vi "02-旋转样品杆控制上位机顺时针归零.vi"() -> ()   [LabVIEW 2017]
uses:
  <vilib>/Instr/_visa.llb/VISA Configure Serial Port (Instr).vi
panel:
  out "逆时针":bool
  out "顺时针":bool
  out "转动角度命令字符串":string
  out "脉冲字符串":string
  out "脉冲数":u32
  out "归零命令字符串":string
  out "频率字符串":string
  out "频率":u32
  in  "停止运动中的电机":bool
  out "转角相对位置":dbl(knob) scale=0.0..360.0
  in  "电机转速设定":dbl(knob)=10.0 min=0.1 max=10.0 scale=0.1..10.0 scale format="%#_2g"
  in  "转动到设定值":bool
  in  "零点归位":bool
  out "样品杆实际值":dbl(slide) scale=-540.0..540.0 scale format="%.2f"
  in  "停止上位机软件系统":bool
  out "波形图表":cluster{"样品杆设定值":dbl, dbl}(graph)
  in  "旋转样品杆控制端口":refnum<visa-resource-name>
  in  "样品杆设定值":dbl(slide) min=-540.0 max=540.0 scale=-540.0..540.0 scale format="%.2g"
  # "旋转样品杆控制测试程序"
  # "转角绝对位置"
  # "样品杆转动位置曲线"
  # "顺时针"
  # "1"
  # "首先要进行零点归位"
  # "逆时针"
  # "转角相对位置"
  # "电机转速设定"
  # "（度/秒）"
  # "（度）"
  # "（度）"
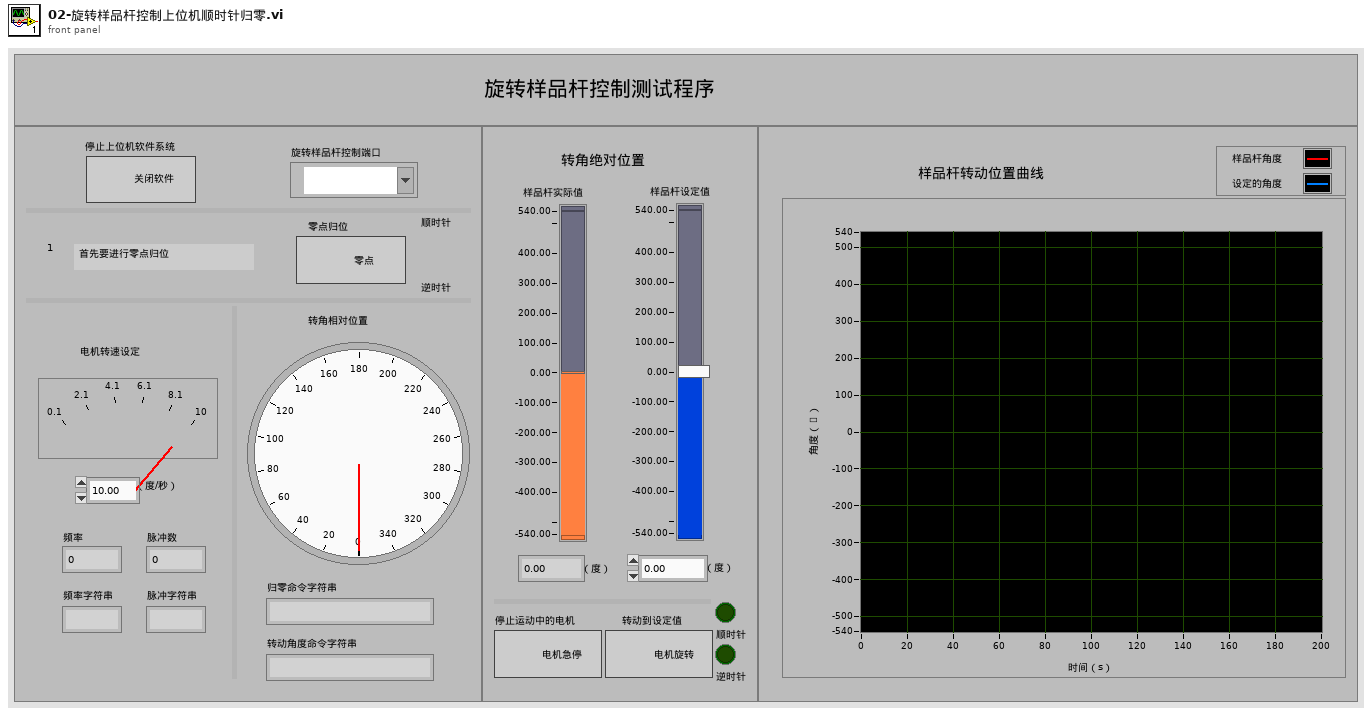
[diagram p1: front panel]
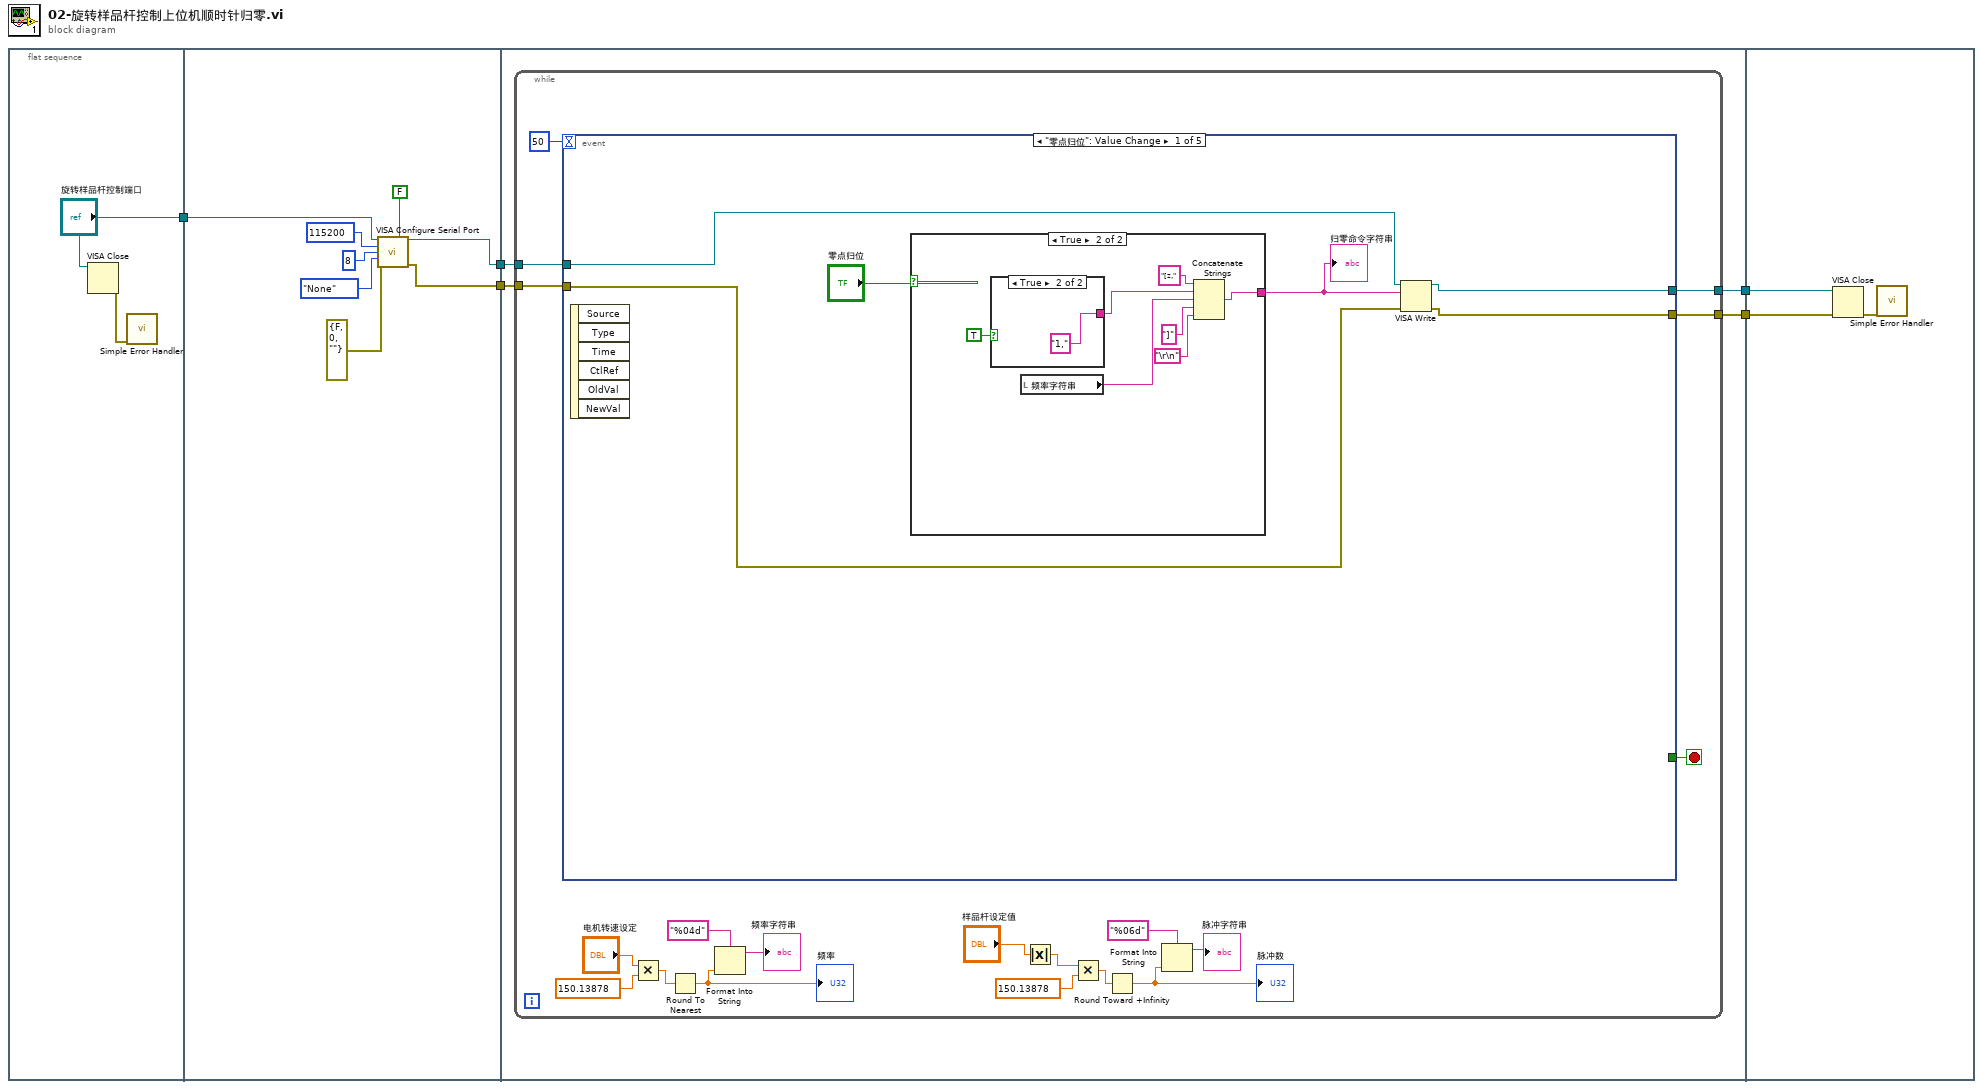
[diagram p0: block diagram]
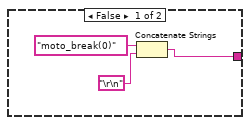
[diagram p2: hidden frame]
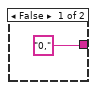
[diagram p3: hidden frame]
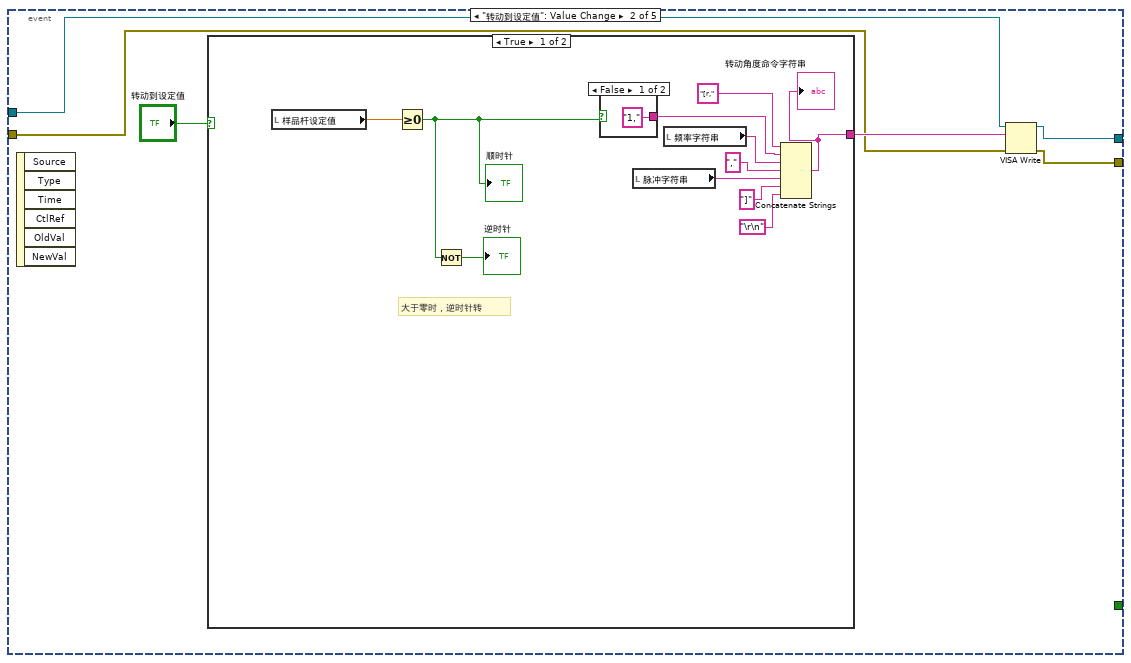
[diagram p4: hidden frame]
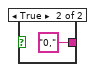
[diagram p5: hidden frame]
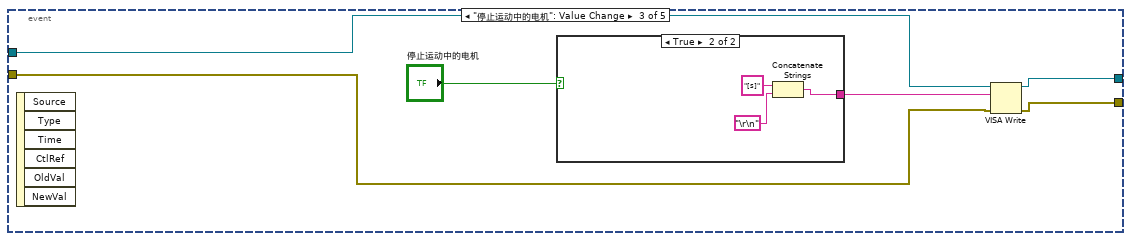
[diagram p7: hidden frame]
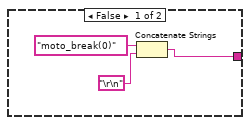
[diagram p8: hidden frame]
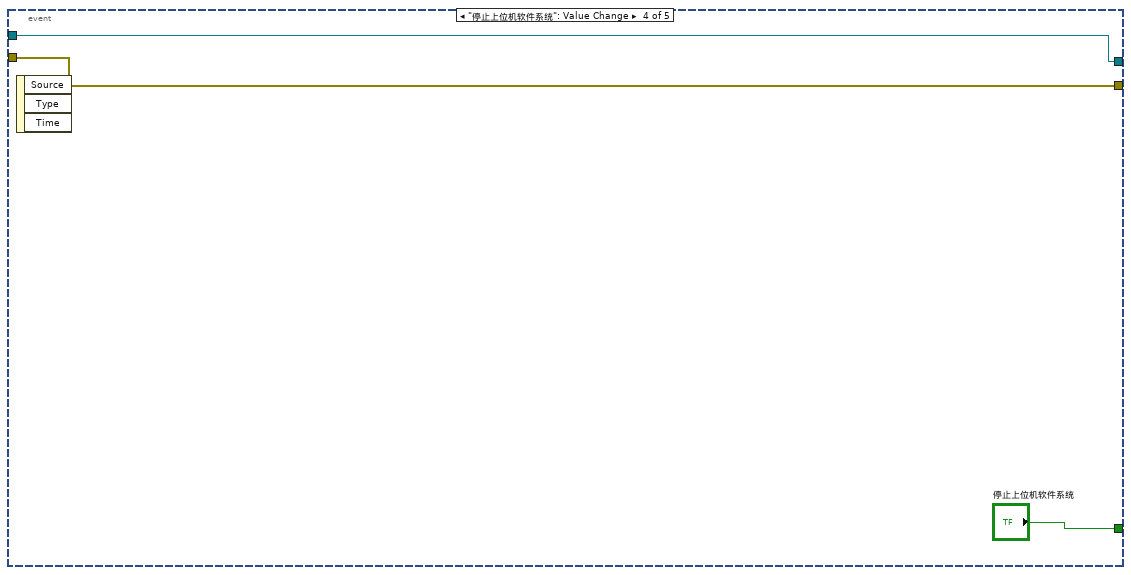
[diagram p9: hidden frame]
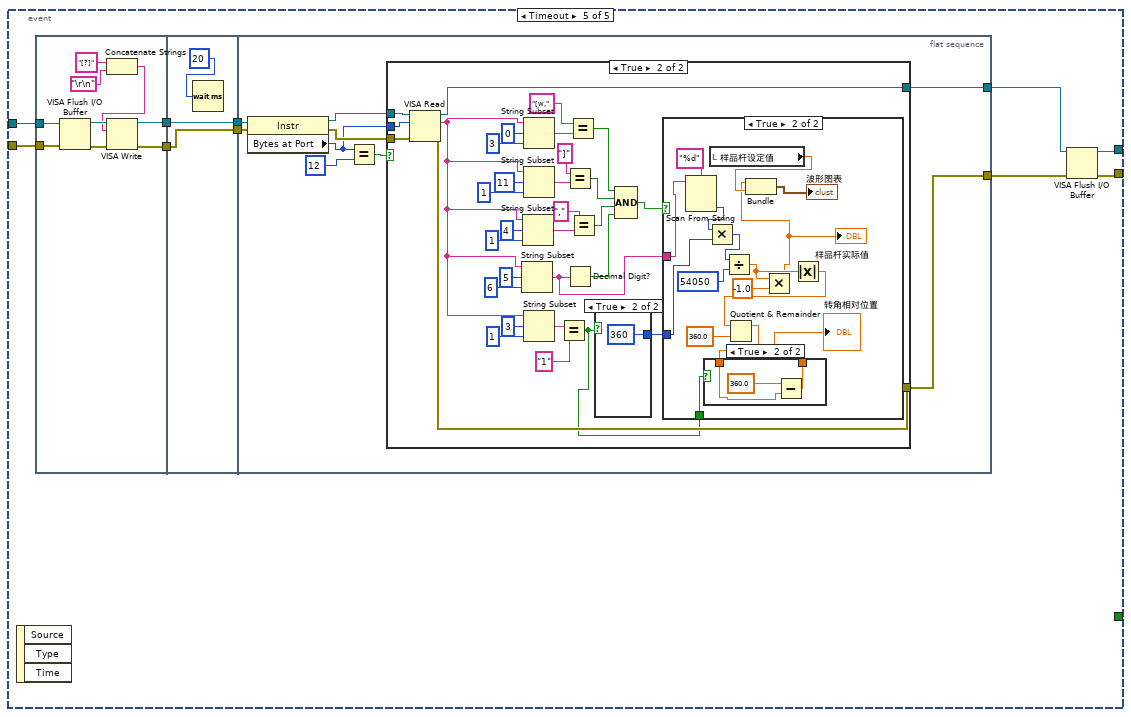
[diagram p10: hidden frame]
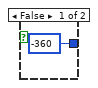
[diagram p12: hidden frame]
diagram:
  n1 = flat-sequence {
    tunnel: ["旋转样品杆控制端口"] -> w1
    tunnel: [w10] -> w3
    tunnel: [w9] -> w2
    tunnel: w1 -> [w8]
    tunnel: [w19] -> w5
    tunnel: [w18] -> w4
    tunnel: w3 -> [w17]
    tunnel: w2 -> [w16]
    tunnel: w5 -> [w180]
    tunnel: w4 -> [w178]
    frame #0 {
      n2 = VISA Close(VISA resource name="旋转样品杆控制端口") -> (error out=w7:errorcluster)  [unwired: 1 in]
      n3 = call <vilib>:"Simple Error Handler.vi"("error in (no error)"=w7) -> ()  [unwired: 4 in, 5 out]
    }
    frame #1 {
      n4 = call-poly "VISA Configure Serial Port"("VISA resource name"=w8, "Enable Termination\nChar (T)"=FALSE ("Enable Termination\nChar (T)"), "baud rate (9600)"=u32 115200, "data bits (8)"=u16 8, "parity (0:none)"=enum16{"None", "Odd", "Even", "Mark", "Space"}."None", "error in (no error)"=errorcluster {"status"=FALSE, "code"=0, "source"=""}) -> ("VISA resource name out"=w10:refnum<visa-resource-name>, "error out"=w9:errorcluster)  [unwired: 8 in]
    }
    frame #2 {
      n5 = while {
        tunnel: [w38] -> w19
        tunnel: [w36] -> w18
        tunnel: w17 -> [w34]
        tunnel: w16 -> [w33]
        stop <- w37 stop-if-true
        n6 = event shown="[0] \"零点归位\": Value Change" {
          selector: _ -> [_ _ _ _ _]
          dyn-events: _ -> [_ _ _ _ _]
          timeout: 50 -> [_ _ _ _ _]
          tunnel: [w44 w57 w76 w89 w100] -> w38
          tunnel: [_ _ _ "停止上位机软件系统" _] -> w37
          tunnel: w34 -> [w41 w61 w79 w88 w98]
          tunnel: w33 -> [w40 w60 w78 w89 w97]
          tunnel: [w43 w58 w77 w88 w99] -> w36
          event "零点归位": Value Change {
            n7 = event-data() -> ()  [unwired: 1 in, 6 out]
            n8 = case shown="True" "零点归位" {
              tunnel: [w45 w53] -> w39
              frame False {
                n9 = Concatenate Strings("moto_break(0)" ("字符串"), "\r\n") -> (w45:string)
              }
              frame True {
                n10 = case shown="True" TRUE {
                  tunnel: ["0," ("字符串") "1," ("字符串")] -> w52
                  frame False {
                  }
                  frame True {
                  }
                }
                n11 = local read "频率字符串"() -> (w49:string)
                n12 = Concatenate Strings("[z," ("字符串"), w52, w49, "]" ("字符串"), "\r\n") -> (w53:string)
              }
            }
            "归零命令字符串" <- w39
            n13 = VISA Write(VISA resource name=w41, write buffer=w39, error in (no error)=w40) -> (VISA resource name out=w43:refnum<visa-resource-name>, error out=w44:errorcluster)  [unwired: 1 out]
          }
          event "转动到设定值": Value Change {
            n14 = event-data() -> ()  [unwired: 1 in, 6 out]
            n15 = case shown="True" "转动到设定值" {
              tunnel: [w68 _] -> w62
              frame True {
                # "大于零时，逆时针转"
                n16 = local read "样品杆设定值"() -> (w65:dbl)
                n17 = Greater Or Equal To 0?(x=w65) -> (x >= 0?=w63:bool)
                "顺时针" <- w63
                n18 = Not(x=w63) -> (.not. x?=→"逆时针":bool)
                n19 = case shown="False" w63 {
                  tunnel: ["1," ("字符串") "0," ("字符串")] -> w67
                  frame False {
                  }
                  frame True {
                  }
                }
                n20 = local read "脉冲字符串"() -> (w69:string)
                n21 = local read "频率字符串"() -> (w73:string)
                n22 = Concatenate Strings("[r,", w67, w73, "," ("字符串"), w69, "]" ("字符串"), "\r\n") -> (w68:string)
                "转动角度命令字符串" <- w68
              }
              frame False {
              }
            }
            n23 = VISA Write(VISA resource name=w61, write buffer=w62, error in (no error)=w60) -> (VISA resource name out=w58:refnum<visa-resource-name>, error out=w57:errorcluster)  [unwired: 1 out]
          }
          event "停止运动中的电机": Value Change {
            n24 = event-data() -> ()  [unwired: 1 in, 6 out]
            n25 = case shown="True" "停止运动中的电机" {
              tunnel: [w82 w85] -> w81
              frame False {
                n26 = Concatenate Strings("moto_break(0)" ("字符串"), "\r\n") -> (w82:string)
              }
              frame True {
                n27 = Concatenate Strings("[s]" ("字符串"), "\r\n") -> (w85:string)
              }
            }
            n28 = VISA Write(VISA resource name=w79, write buffer=w81, error in (no error)=w78) -> (VISA resource name out=w77:refnum<visa-resource-name>, error out=w76:errorcluster)  [unwired: 1 out]
          }
          event "停止上位机软件系统": Value Change {
            n29 = event-data() -> ()  [unwired: 1 in, 3 out]
          }
          event Timeout {
            n30 = event-data() -> ()  [unwired: 1 in, 3 out]
            n31 = flat-sequence {
              tunnel: w98 -> [w104]
              tunnel: w97 -> [w103]
              tunnel: [w102] -> w95
              tunnel: [w101] -> w93
              tunnel: [w111] -> w96
              tunnel: w95 -> [w111]
              tunnel: [w110] -> w94
              tunnel: w93 -> [w110]
              tunnel: w96 -> [w121]
              tunnel: w94 -> [w120]
              tunnel: [w114] -> w92
              tunnel: [w113] -> w91
              frame #0 {
                n32 = VISA Flush I/O Buffer(VISA resource name=w104, error in (no error)=w103) -> (VISA resource name out=w108:refnum<visa-resource-name>, error out=w109:errorcluster)  [unwired: 1 in]
                n33 = Concatenate Strings("[?]" ("字符串"), "\r\n") -> (w105:string)
                n34 = VISA Write(VISA resource name=w108, write buffer=w105, error in (no error)=w109) -> (VISA resource name out=w102:refnum<visa-resource-name>, error out=w101:errorcluster)  [unwired: 1 out]
              }
              frame #1 {
                n35 = Wait (ms)(milliseconds to wait=u32 20 ("等待时间（毫秒）")) -> ()  [unwired: 1 out]
              }
              frame #2 {
                n36 = property class="Instr"(reference=w121, error in=w120) -> (reference out=w116:refnum<visa-resource-name>, error out=w117:errorcluster, "Bytes at Port"=w115:u32)
                n37 = Equal?(x=w115, y=u32 12) -> (x = y?=w118:bool)
                n38 = case shown="True" w118 {
                  tunnel: w117 -> [w122 w155]
                  tunnel: w116 -> [w123 w154]
                  tunnel: w115 -> [_ w153]
                  tunnel: [w123 w133] -> w114
                  tunnel: [w122 w132] -> w113
                  frame False {
                  }
                  frame True {
                    n39 = VISA Read(VISA resource name=w154, byte count=w153, error in (no error)=w155) -> (VISA resource name out=w133:refnum<visa-resource-name>, read buffer=w130:string, error out=w132:errorcluster)  [unwired: 1 out]
                    n40 = String Subset(string=w130, offset (0)=5 ("偏移量(0)"), length (rest)=6 ("长度（剩余）")) -> (substring=w131:string)
                    n41 = String Subset(string=w130, offset (0)=4 ("偏移量(0)"), length (rest)=1 ("长度（剩余）")) -> (substring=w147:string)
                    n42 = String Subset(string=w130, offset (0)=0 ("偏移量(0)"), length (rest)=3 ("长度（剩余）")) -> (substring=w143:string)
                    n43 = String Subset(string=w130, offset (0)=11 ("偏移量(0)"), length (rest)=1 ("长度（剩余）")) -> (substring=w145:string)
                    n44 = String Subset(string=w130, offset (0)=3 ("偏移量(0)"), length (rest)=1 ("长度（剩余）")) -> (substring=w125:string)
                    n45 = Equal?(x=w125, y="1") -> (x = y?=w124:bool)
                    n46 = Equal?(x="]", y=w145) -> (x = y?=w150:bool)
                    n47 = Decimal Digit?(1:w131) -> (0:w152:bool)
                    n48 = Equal?(x="[w,", y=w143) -> (x = y?=w149:bool)
                    n49 = Equal?(x=",", y=w147) -> (x = y?=w151:bool)
                    n50 = case shown="True" w124 {
                      tunnel: [-360 ("y") 360 ("y")] -> w126
                      frame False {
                      }
                      frame True {
                      }
                    }
                    n51 = Compound Arithmetic op=AND(w149, w150, w151, w152) -> (w134:bool)
                    n52 = case shown="True" w134 {
                      tunnel: w131 -> [_ w168]
                      tunnel: w126 -> [_ w163]
                      tunnel: w124 -> [_ w162]
                      frame False {
                      }
                      frame True {
                        n53 = Scan From String(format string="%d" ("格式字符串"), input string=w168) -> (output 1=w167:i32)  [unwired: 3 in, 3 out]
                        n54 = Multiply(x=w167, y=w163) -> (x*y=w172:i32)
                        n55 = local read "样品杆设定值"() -> (w170:dbl)
                        n56 = Divide(x=w172, y=54050) -> (x/y=w164:dbl)
                        n57 = Multiply(x=w164, y=-1.0) -> (x*y=w158:dbl)
                        "样品杆实际值" <- w158
                        n58 = Bundle(w158, "样品杆设定值"=w170) -> (→"波形图表":cluster{dbl, "样品杆设定值":dbl})  [unwired: 1 in]
                        n59 = Absolute Value(x=w164) -> (abs(x)=w165:dbl)
                        n60 = Quotient & Remainder(x=w165, y=360.0) -> (x-y*floor(x/y)=w160:dbl)  [unwired: 1 out]
                        n61 = case shown="True" w162 {
                          tunnel: [w174 w177] -> w161
                          tunnel: w160 -> [w174 w175]
                          frame False {
                          }
                          frame True {
                            n62 = Subtract(x=360.0, y=w175) -> (x-y=w177:dbl)
                          }
                        }
                        "转角相对位置" <- w161
                      }
                    }
                  }
                }
              }
            }
            n63 = VISA Flush I/O Buffer(VISA resource name=w92, error in (no error)=w91) -> (VISA resource name out=w99:refnum<visa-resource-name>, error out=w100:errorcluster)  [unwired: 1 in]
          }
        }
        n64 = Multiply(x="电机转速设定", y=150.13878) -> (x*y=w31:dbl)
        n65 = Round To Nearest(number=w31) -> (nearest integer value=w27:dbl)
        "频率" <- w27
        n66 = Format Into String(format string="%04d" ("格式字符串"), w27) -> (resulting string=→"频率字符串":string)  [unwired: 2 in, 1 out]
        n67 = Absolute Value(x="样品杆设定值") -> (abs(x)=w20:dbl)
        n68 = Multiply(x=w20, y=150.13878) -> (x*y=w23:dbl)
        n69 = Round Toward +Infinity(x=w23) -> (ceil(x): smallest int >= x=w25:dbl)
        "脉冲数" <- w25
        n70 = Format Into String(format string="%06d" ("格式字符串"), w25) -> (resulting string=→"脉冲字符串":string)  [unwired: 2 in, 1 out]
      }
    }
    frame #3 {
      n71 = VISA Close(VISA resource name=w178, error in (no error)=w180) -> (error out=w179:errorcluster)
      n72 = call <vilib>:"Simple Error Handler.vi"("error in (no error)"=w179) -> ()  [unwired: 4 in, 5 out]
    }
  }
